vi "Run.vi"(11 "Audio Data":refnum<queue>) -> ()   [LabVIEW 2020, in "Audio Recording.lvlib"]
uses:
  Audio Recording.lvlib
  Audio Output/Audio Output Queue Type.ctl
  <vilib>/sound2/lvsound2.llb/Sound File Refnum.ctl
  <vilib>/sound2/lvsound2.llb/Sound Data Format.ctl
  <vilib>/sound2/lvsound2.llb/Sound File Write Open.vi
  <vilib>/sound2/lvsound2.llb/Sound File Write (I16).vi
  Audio Output/Audio Output.lvlib
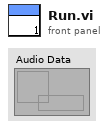
[diagram p1: front panel]
types:
  T1 = typedef "Sound File Refnum.ctl" = refnum<file>
  T2 = typedef "Sound Data Format.ctl" = cluster{"sample rate (S/s)":dbl, "number of channels":i32, "bits per sample":i32}
  T3 = typedef "Audio Output.lvlib/Audio Output Queue Type.ctl" = cluster{"Master":waveform(i16)[], "Headphones":waveform(i16)[], "Start Time":dbl, "Record":bool}
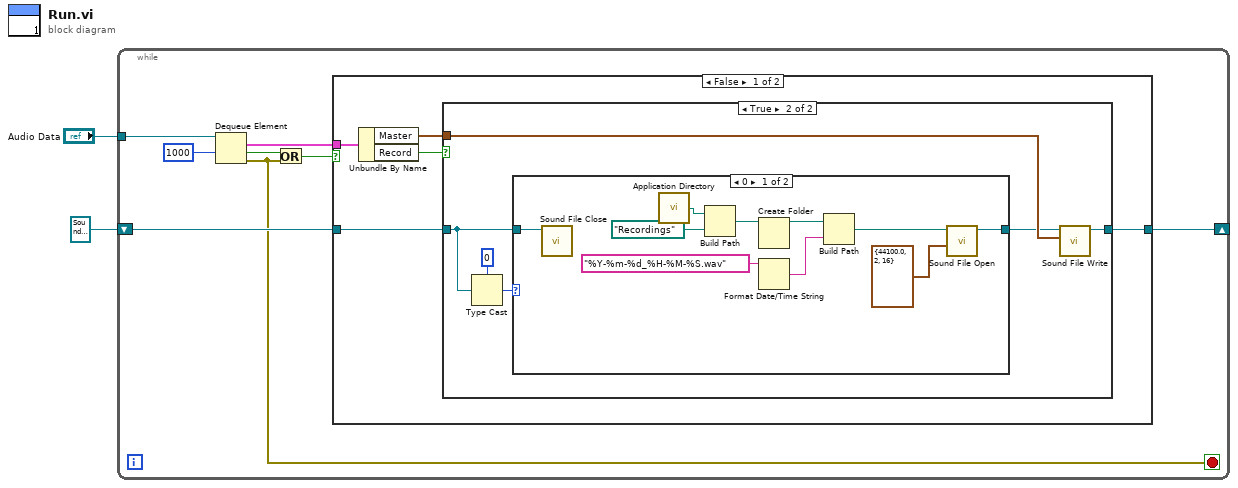
[diagram p0: block diagram]
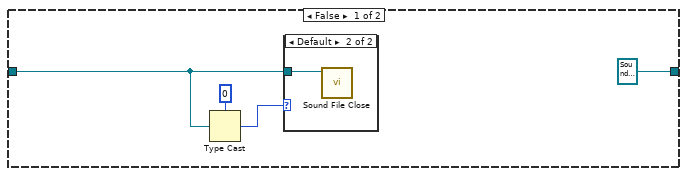
[diagram p2: hidden frame]
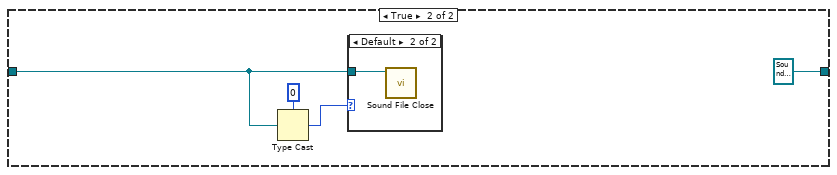
[diagram p5: hidden frame]
diagram:
  n1 = while {
    tunnel: "Audio Data" -> [w10]
    shift-right: [w7] -> _
    shift-left: T1 refnum ("sound file refnum out") -> [w8]
    stop <- w4 stop-if-true
    n2 = Dequeue Element(queue=w10, timeout in ms (-1)=1000) -> (element=w9:T3, timed out?=w6:bool, error out=w4:errorcluster)  [unwired: 1 in, 1 out]
    n3 = Or(x=w6, y=w4) -> (x .or. y?=w5:bool)
    n4 = case shown="False" w5 {
      tunnel: w9 -> [w15 _]
      tunnel: w8 -> [w13 w39]
      tunnel: [w12 T1 refnum ("sound file refnum out")] -> w7
      frame False {
        n5 = Unbundle By Name(w15) -> ("Master"=w14:waveform(i16)[], "Record"=w11:bool)
        n6 = case shown="True" w11 {
          tunnel: w14 -> [_ w26]
          tunnel: w13 -> [w17 w23]
          tunnel: [T1 refnum ("sound file refnum out") w24] -> w12
          frame False {
            n7 = Type Cast(type=0, x=w17) -> (*(type *) &x=w16:i32)
            n8 = case shown="Default" w16 {
              tunnel: w17 -> [_ w20]
              frame 0 {
              }
              frame Default {
                n9 = call <vilib>:"Sound File Close.vi"("sound file refnum"=w20) -> ()  [unwired: 10 in, 1 out]
              }
            }
          }
          frame True {
            n10 = Type Cast(type=0, x=w23) -> (*(type *) &x=w21:i32)
            n11 = case shown="0" w21 {
              tunnel: [w28 w37] -> w25
              tunnel: w23 -> [w27 w37]
              frame 0 {
                n12 = call <vilib>:"Sound File Close.vi"("sound file refnum"=w27) -> ()  [unwired: 10 in, 1 out]
                n13 = call <vilib>:"Application Directory.vi"() -> ("Application Directory"=w33:path)
                n14 = Build Path(base path=w33, name or relative path=path "Recordings") -> (appended path=w34:path)
                n15 = Create Folder(path (use dialog)=w34) -> (created path=w31:path)  [unwired: 2 in, 2 out]
                n16 = Format Date/Time String(time format string (%c)="%Y-%m-%d_%H-%M-%S.wav") -> (date/time string=w30:string)  [unwired: 2 in]
                n17 = Build Path(base path=w31, name or relative path=w30) -> (appended path=w29:path)
                n18 = call-poly <vilib>:"Sound File Open.vi"("sound format"=T2 {"sample rate (S/s)"=44100.0, "number of channels"=2, "bits per sample"=16}, "path"=w29) -> ("sound file refnum"=w28:T1)  [unwired: 8 in, 1 out]
              }
              frame Default {
              }
            }
            n19 = call-poly <vilib>:"Sound File Write.vi"("data"=w26, "sound file refnum"=w25) -> ("sound file refnum out"=w24:T1)  [unwired: 8 in, 1 out]
          }
        }
      }
      frame True {
        n20 = Type Cast(type=0, x=w39) -> (*(type *) &x=w38:i32)
        n21 = case shown="Default" w38 {
          tunnel: w39 -> [_ w42]
          frame 0 {
          }
          frame Default {
            n22 = call <vilib>:"Sound File Close.vi"("sound file refnum"=w42) -> ()  [unwired: 10 in, 1 out]
          }
        }
      }
    }
  }
